vi "Configure Dialog.vi"(8 "error in (no error)":errorcluster, 11 "Display WebPubURL Msg.lvclass":refnum<class "Display WebPubURL Msg.lvclass">) -> (0 "error out":errorcluster, 2 "Ok?":bool, 3 "Display WebPubURL Msg.lvclass":refnum<class "Display WebPubURL Msg.lvclass">)   [LabVIEW 2016, in "CS++BaseActor.lvlib" / "Display WebPubURL Msg.lvclass"]
uses:
  Display WebPubURL Msg.lvclass
panel:
  in  "Cancel Button":bool
  in  "OK Button":bool
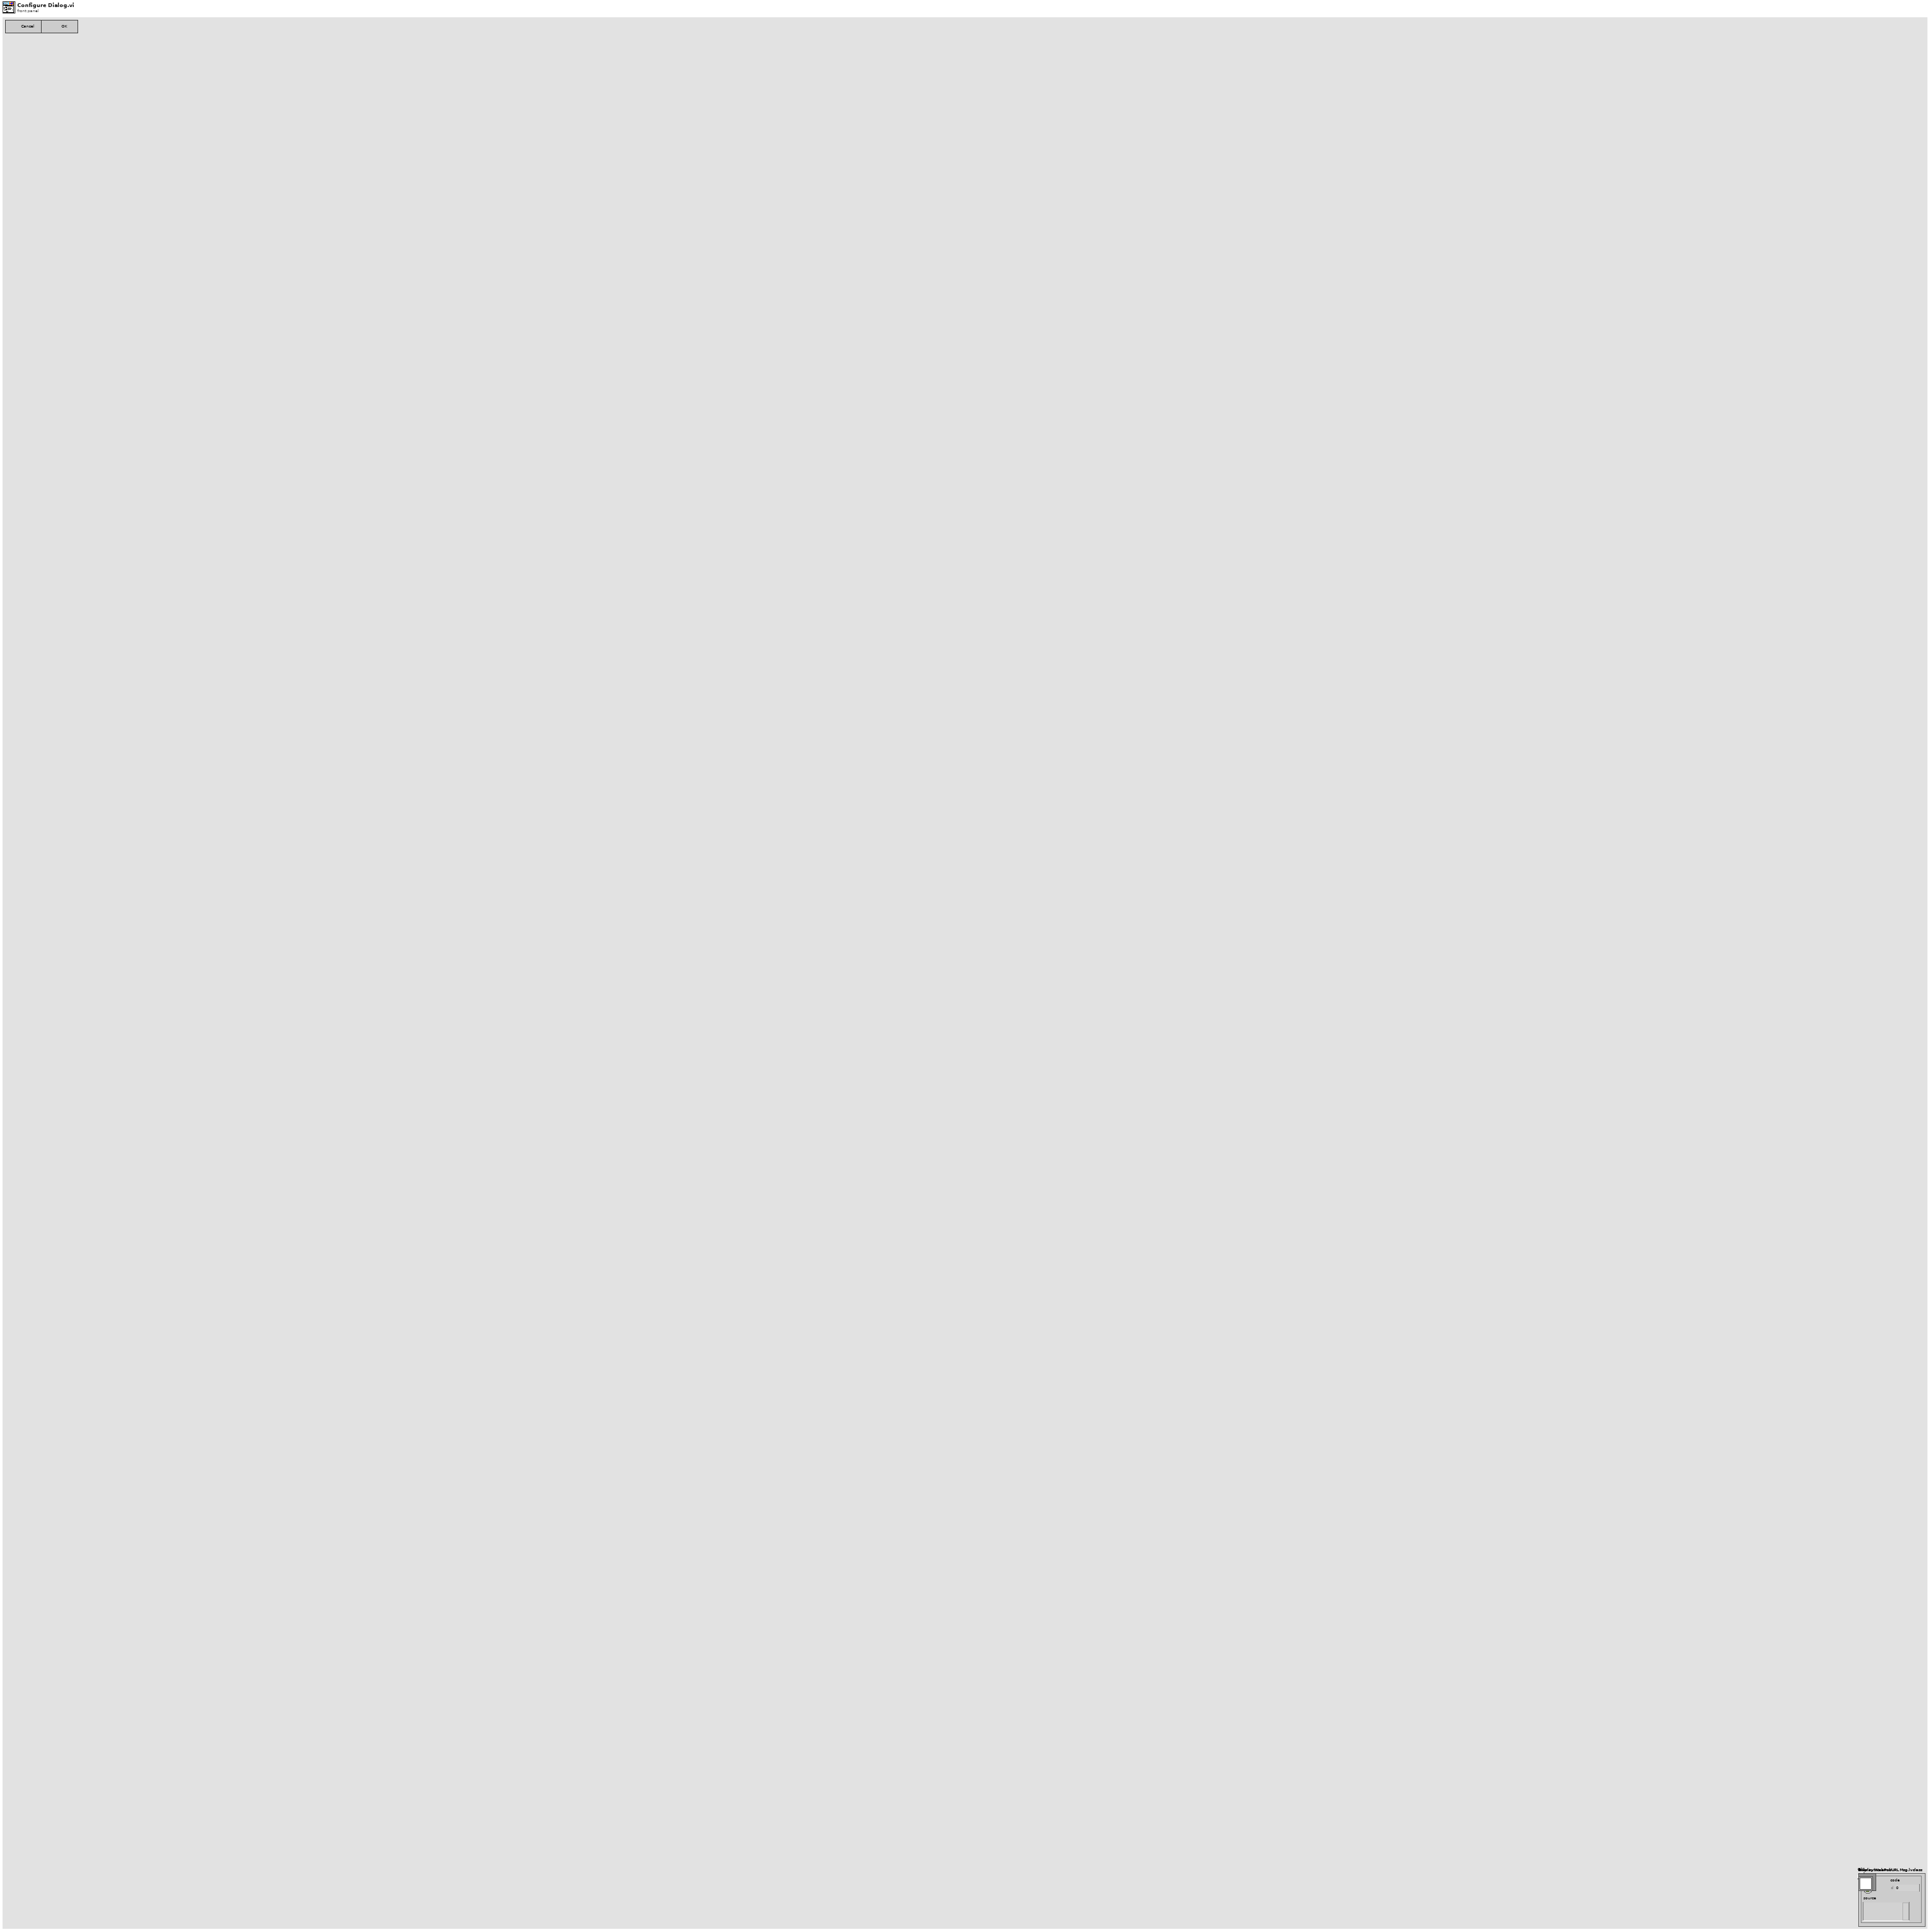
[diagram p1: front panel]
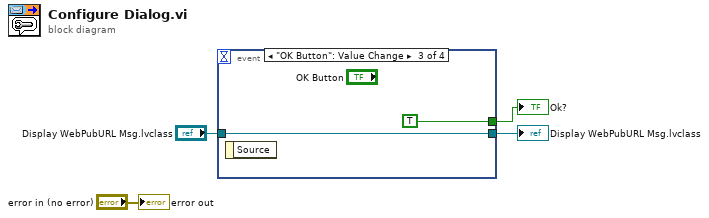
[diagram p0: block diagram]
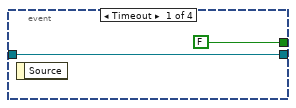
[diagram p2: hidden frame]
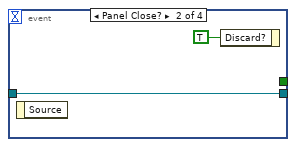
[diagram p3: hidden frame]
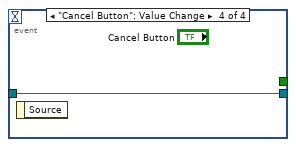
[diagram p4: hidden frame]
diagram:
  n1 = event shown="[2] \"OK Button\": Value Change" {
    selector: _ -> [_ _ _ _]
    dyn-events: _ -> [_ _ _ _]
    timeout: _ -> [_ _ _ _]
    tunnel: [w5 w7 w10 w11] -> w2
    tunnel: "Display WebPubURL Msg.lvclass" -> [w5 w7 w10 w11]
    tunnel: [FALSE _ TRUE _] -> w3
    event Timeout {
      n2 = event-data() -> ()  [unwired: 1 in, 1 out]
    }
    event Panel Close? {
      n3 = event-data() -> ()  [unwired: 1 in, 1 out]
      n4 = event-data ("Event Filter Node")("Discard?"=TRUE) -> ()  [unwired: 1 in, 1 out]
    }
    event "OK Button": Value Change {
      n5 = event-data() -> ()  [unwired: 1 in, 1 out]
    }
    event "Cancel Button": Value Change {
      n6 = event-data() -> ()  [unwired: 1 in, 1 out]
    }
  }
  "Ok?" <- w3
  "Display WebPubURL Msg.lvclass" <- w2
  "error out" <- "error in (no error)"
